vi "Reset.vi"(11 "handler in":refnum<class "Formatting Handler.lvclass">) -> (2 "successful?":bool, 3 "handler out":refnum<class "Formatting Handler.lvclass">)   [LabVIEW 2024, in "Logging.lvlib" / "Formatting Handler.lvclass"]
uses:
  Formatting Handler.lvclass
  Formatting Handler.lvclass/Formatting Handler.ctl
panel:
  # "Connector Pane"
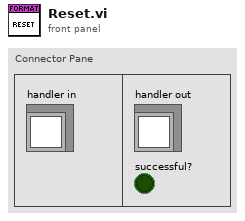
[diagram p1: front panel]
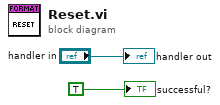
[diagram p0: block diagram]
diagram:
  "handler out" <- "handler in"
  "successful?" <- TRUE ("successful?")
